vi "Initiate Model and Serial Numbers.vi"(8 "error in (no error)":errorcluster, 9 "Serial CmbBox Ref":refnum<vi>, 10 "Model CmbBox Ref":refnum<vi>, 11 "Database in":refnum<queue>) -> (0 "error out":errorcluster, 3 "Database out":refnum<queue>)   [LabVIEW 2026, in "Analysis.lvlib"]
uses:
  Analysis.lvlib
  support/Architecture/Message Queue/Message Cluster.ctl
  controls/UI/UI List Type.ctl
  controls/UI/UI Device Type.ctl
  controls/UI/Measurement Role.ctl
  Settings/Settings.lvlib
  support/Architecture/Message Queue/Message Queue.lvlib
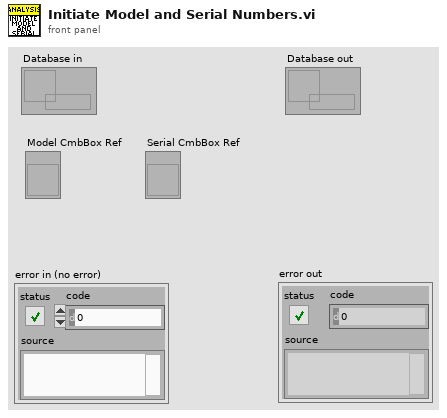
[diagram p1: front panel]
types:
  T1 = typedef "Settings.lvlib/Measurement Role.ctl" = enum16{"Controller", "Reference", "UUT", "Disable", "All"}
  T2 = typedef "Settings.lvlib/UI Device Type.ctl" = enum16{"Measurement", "Controller"}
  T3 = typedef "UI List Type.ctl" = enum16{"Model Numbers", "Serial Numbers", "Operators", "Calibration Points", "Start Run Times"}
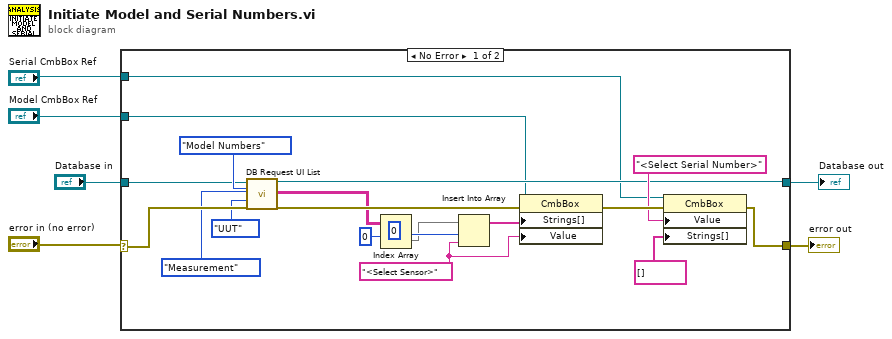
[diagram p0: block diagram]
diagram:
  n1 = case shown="No Error" "error in (no error)" {
    selector: "error in (no error)" -> [w13 w27]
    tunnel: [w12 w27] -> w6
    tunnel: "Database in" -> [w17 w26]
    tunnel: [w16 w26] -> w4
    tunnel: "Serial CmbBox Ref" -> [w15 _]
    tunnel: "Model CmbBox Ref" -> [w14 _]
    frame No Error {
      w23 = "<Select Sensor>"
      n2 = call "DB Request UI List.vi"("Database in"=w17, "UI List Type"=UI_List_Type."Model Numbers", "UI Device Type"=UI_Device_Type."Measurement", "Measurement Role"=Measurement_Role."UUT", "error in (no error)"=w13) -> ("Database out"=w16:refnum<queue>, "Results"=w11:string[][], "error out"=w21:errorcluster)  [unwired: 12 in]
      n3 = Index Array(array=w11, index (row)=0) -> (element=w9:string[])  [unwired: 1 in]
      n4 = Insert Into Array(array=w9, index=0, new element=w23) -> (w24:string[])
      n5 = property on="Property Node" class="CmbBox"(reference=w14, error in=w21, "Strings[]"=w24, "Value"=w23) -> (error out=w25:errorcluster)  [unwired: 1 out]
      n6 = property on="Property Node" class="CmbBox"(reference=w15, error in=w25, "Value"="<Select Serial Number>", "Strings[]"=string[] [] ("Strings []")) -> (error out=w12:errorcluster)  [unwired: 1 out]
    }
    frame Error {
    }
  }
  "error out" <- w6
  "Database out" <- w4
